vi "点对点.vi"(1 "错误输入":errorcluster, 2 "目标位置":cluster{"x（cm）":dbl, "y（cm）":dbl, "角度（度）":dbl}, 3 "I/O":T11) -> (0 "错误输出":errorcluster)   [LabVIEW 2016]
uses:
  <vilib>/myRIO/Instrument Drivers/Onboard IO/PWM/typedefs/PWM Reference.ctl
  <vilib>/myRIO/Common/Instrument Driver Framework/Utilities/typedefs/myRIO Generic Hardware Reference.ctl
  <vilib>/myRIO/Common/Instrument Driver Framework/Utilities/typedefs/Hardware Version Enum.ctl
  <vilib>/myRIO/Common/Instrument Driver Framework/Utilities/typedefs/myRIO v1.0 Reference.ctl
  <vilib>/myRIO/Common/Instrument Driver Framework/Utilities/typedefs/Generic FPGA Reference.ctl
  <vilib>/myRIO/Common/Instrument Driver Framework/myRIO v1.0/PWM/typedefs/PWM Channels Enum.ctl
  <vilib>/myRIO/Instrument Drivers/Onboard IO/PWM/typedefs/PWM Configuration.ctl
  <vilib>/myRIO/Instrument Drivers/Onboard IO/DIO/typedefs/DIO Reference.ctl
  <vilib>/myRIO/Common/Instrument Driver Framework/myRIO v1.0/DIO/typedefs/DIO Channels List.ctl
  <vilib>/myRIO/Common/Instrument Driver Framework/myRIO v1.0/DIO/typedefs/DIO Channels Enum.ctl
  <vilib>/myRIO/Instrument Drivers/Onboard IO/DIO/DIO.lvlib
  <vilib>/myRIO/Instrument Drivers/Onboard IO/PWM/PWM.lvlib
panel:
  out "前进二":bool
  out "旋转三":bool
  out "旋转二":bool
  out "前进一":bool
  out "速度":dbl[](array[numeric])
  out "旋转一":bool
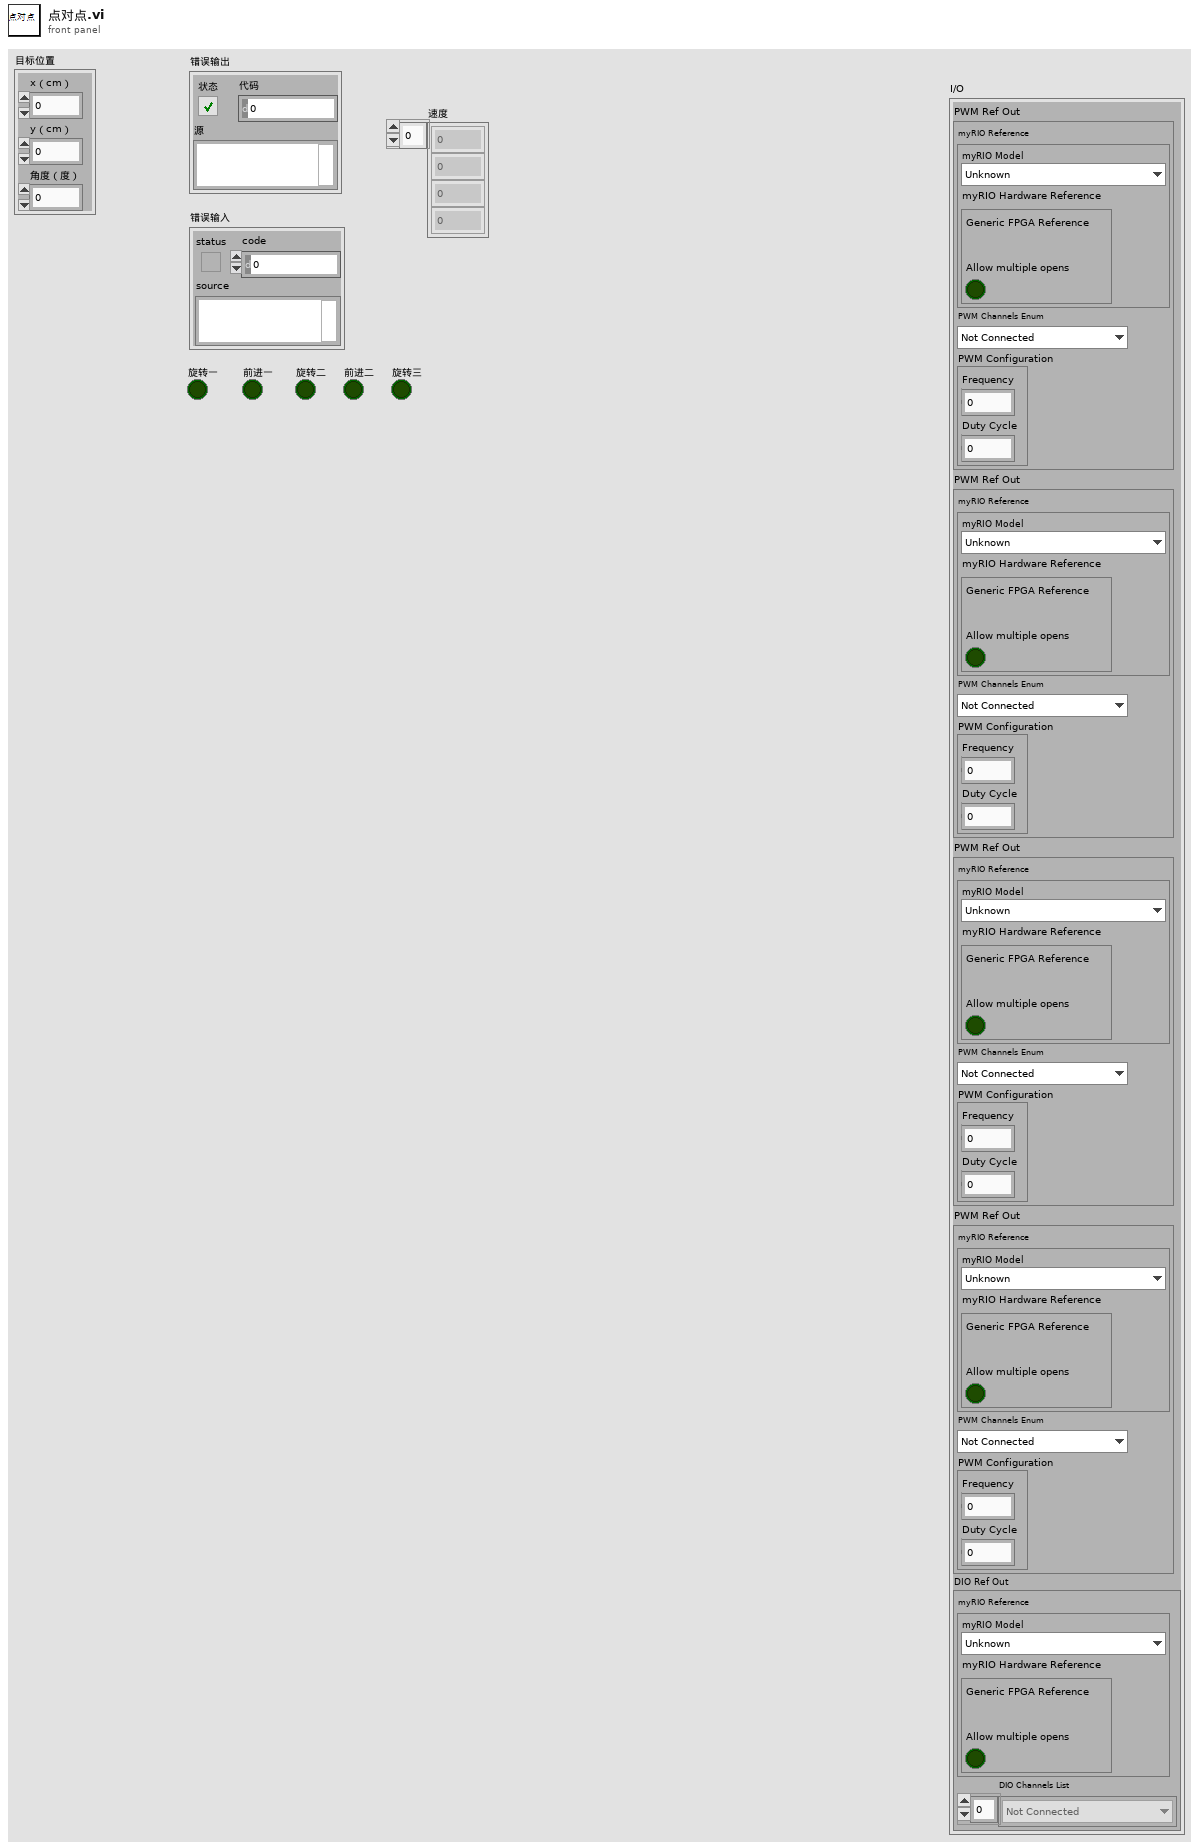
[diagram p1: front panel]
types:
  T1 = typedef "PWM.lvlib/PWM Reference.ctl" = cluster{"myRIO Reference":T2, "PWM Channels Enum":T6, "PWM Configuration":T7}
  T2 = typedef "myRIO Generic Hardware Reference.ctl" = cluster{"myRIO Model":T3, "myRIO Hardware Reference":T4}
  T3 = typedef "Hardware Version Enum.ctl" = enum16{"Unknown", "myRIO-1900", "myRIO-1950", "roboRIO", "NI ELVIS RIO CM"}
  T4 = typedef "myRIO v1.0 Reference.ctl" = cluster{"Generic FPGA Reference":T5, "Allow multiple opens":bool}
  T5 = typedef "Generic FPGA Reference.ctl" = refnum<k20>
  T6 = typedef "PWM Channels Enum.ctl" = enum16{"Not Connected", "C/PWM0", "C/PWM1", "A/PWM0", "A/PWM1", "A/PWM2", "B/PWM0", "B/PWM1", "B/PWM2", "PWM/PWM0", "PWM/PWM1", "PWM/PWM2", "PWM/PWM3", "PWM/PWM4", "PWM/PWM5", "PWM/PWM6", "PWM/PWM7", "PWM/PWM8", "PWM/PWM9"}
  T7 = typedef "PWM.lvlib/PWM Configuration.ctl" = cluster{"Frequency":dbl, "Duty Cycle":dbl}
  T8 = typedef "DIO.lvlib/DIO Reference.ctl" = cluster{"myRIO Reference":T2, "DIO Channels List":T9}
  T9 = typedef "DIO Channels List.ctl" = T10[]
  T10 = typedef "DIO Channels Enum.ctl" = enum16{"Not Connected", "C/DIO0", "C/DIO1", "C/DIO2", "C/DIO3", "C/DIO4", "C/DIO5", "C/DIO6", "C/DIO7", "A/DIO0", "A/DIO1", "A/DIO2", "A/DIO3", "A/DIO4", "A/DIO5", "A/DIO6", "A/DIO7", "A/DIO8", "A/DIO9", "A/DIO10", "A/DIO11", "A/DIO12", "A/DIO13", "A/DIO14", "A/DIO15", "B/DIO0", "B/DIO1", "B/DIO2", "B/DIO3", "B/DIO4", "B/DIO5", "B/DIO6", "B/DIO7", "B/DIO8", "B/DIO9", "B/DIO10", "B/DIO11", "B/DIO12", "B/DIO13", "B/DIO14", "B/DIO15", "LED0", "LED1", "LED2", "LED3", "Button0", "DIO/DIO0", "DIO/DIO1", "DIO/DIO2", "DIO/DIO3", "DIO/DIO4", "DIO/DIO5", "DIO/DIO6", "DIO/DIO7", "DIO/DIO8", "DIO/DIO9", "SPI/CS0", "SPI/CS1", "SPI/CS2", "SPI/CS3", "LED RADIO (Green)", "LED RADIO (Red)", "LED COMM (Green)", "LED COMM (Red)", "LED MODE (Green)", "LED MODE (Red)"}
  T11 = cluster{"PWM Ref Out":T1, "PWM Ref Out":T1, "PWM Ref Out":T1, "PWM Ref Out":T1, "DIO Ref Out":T8}
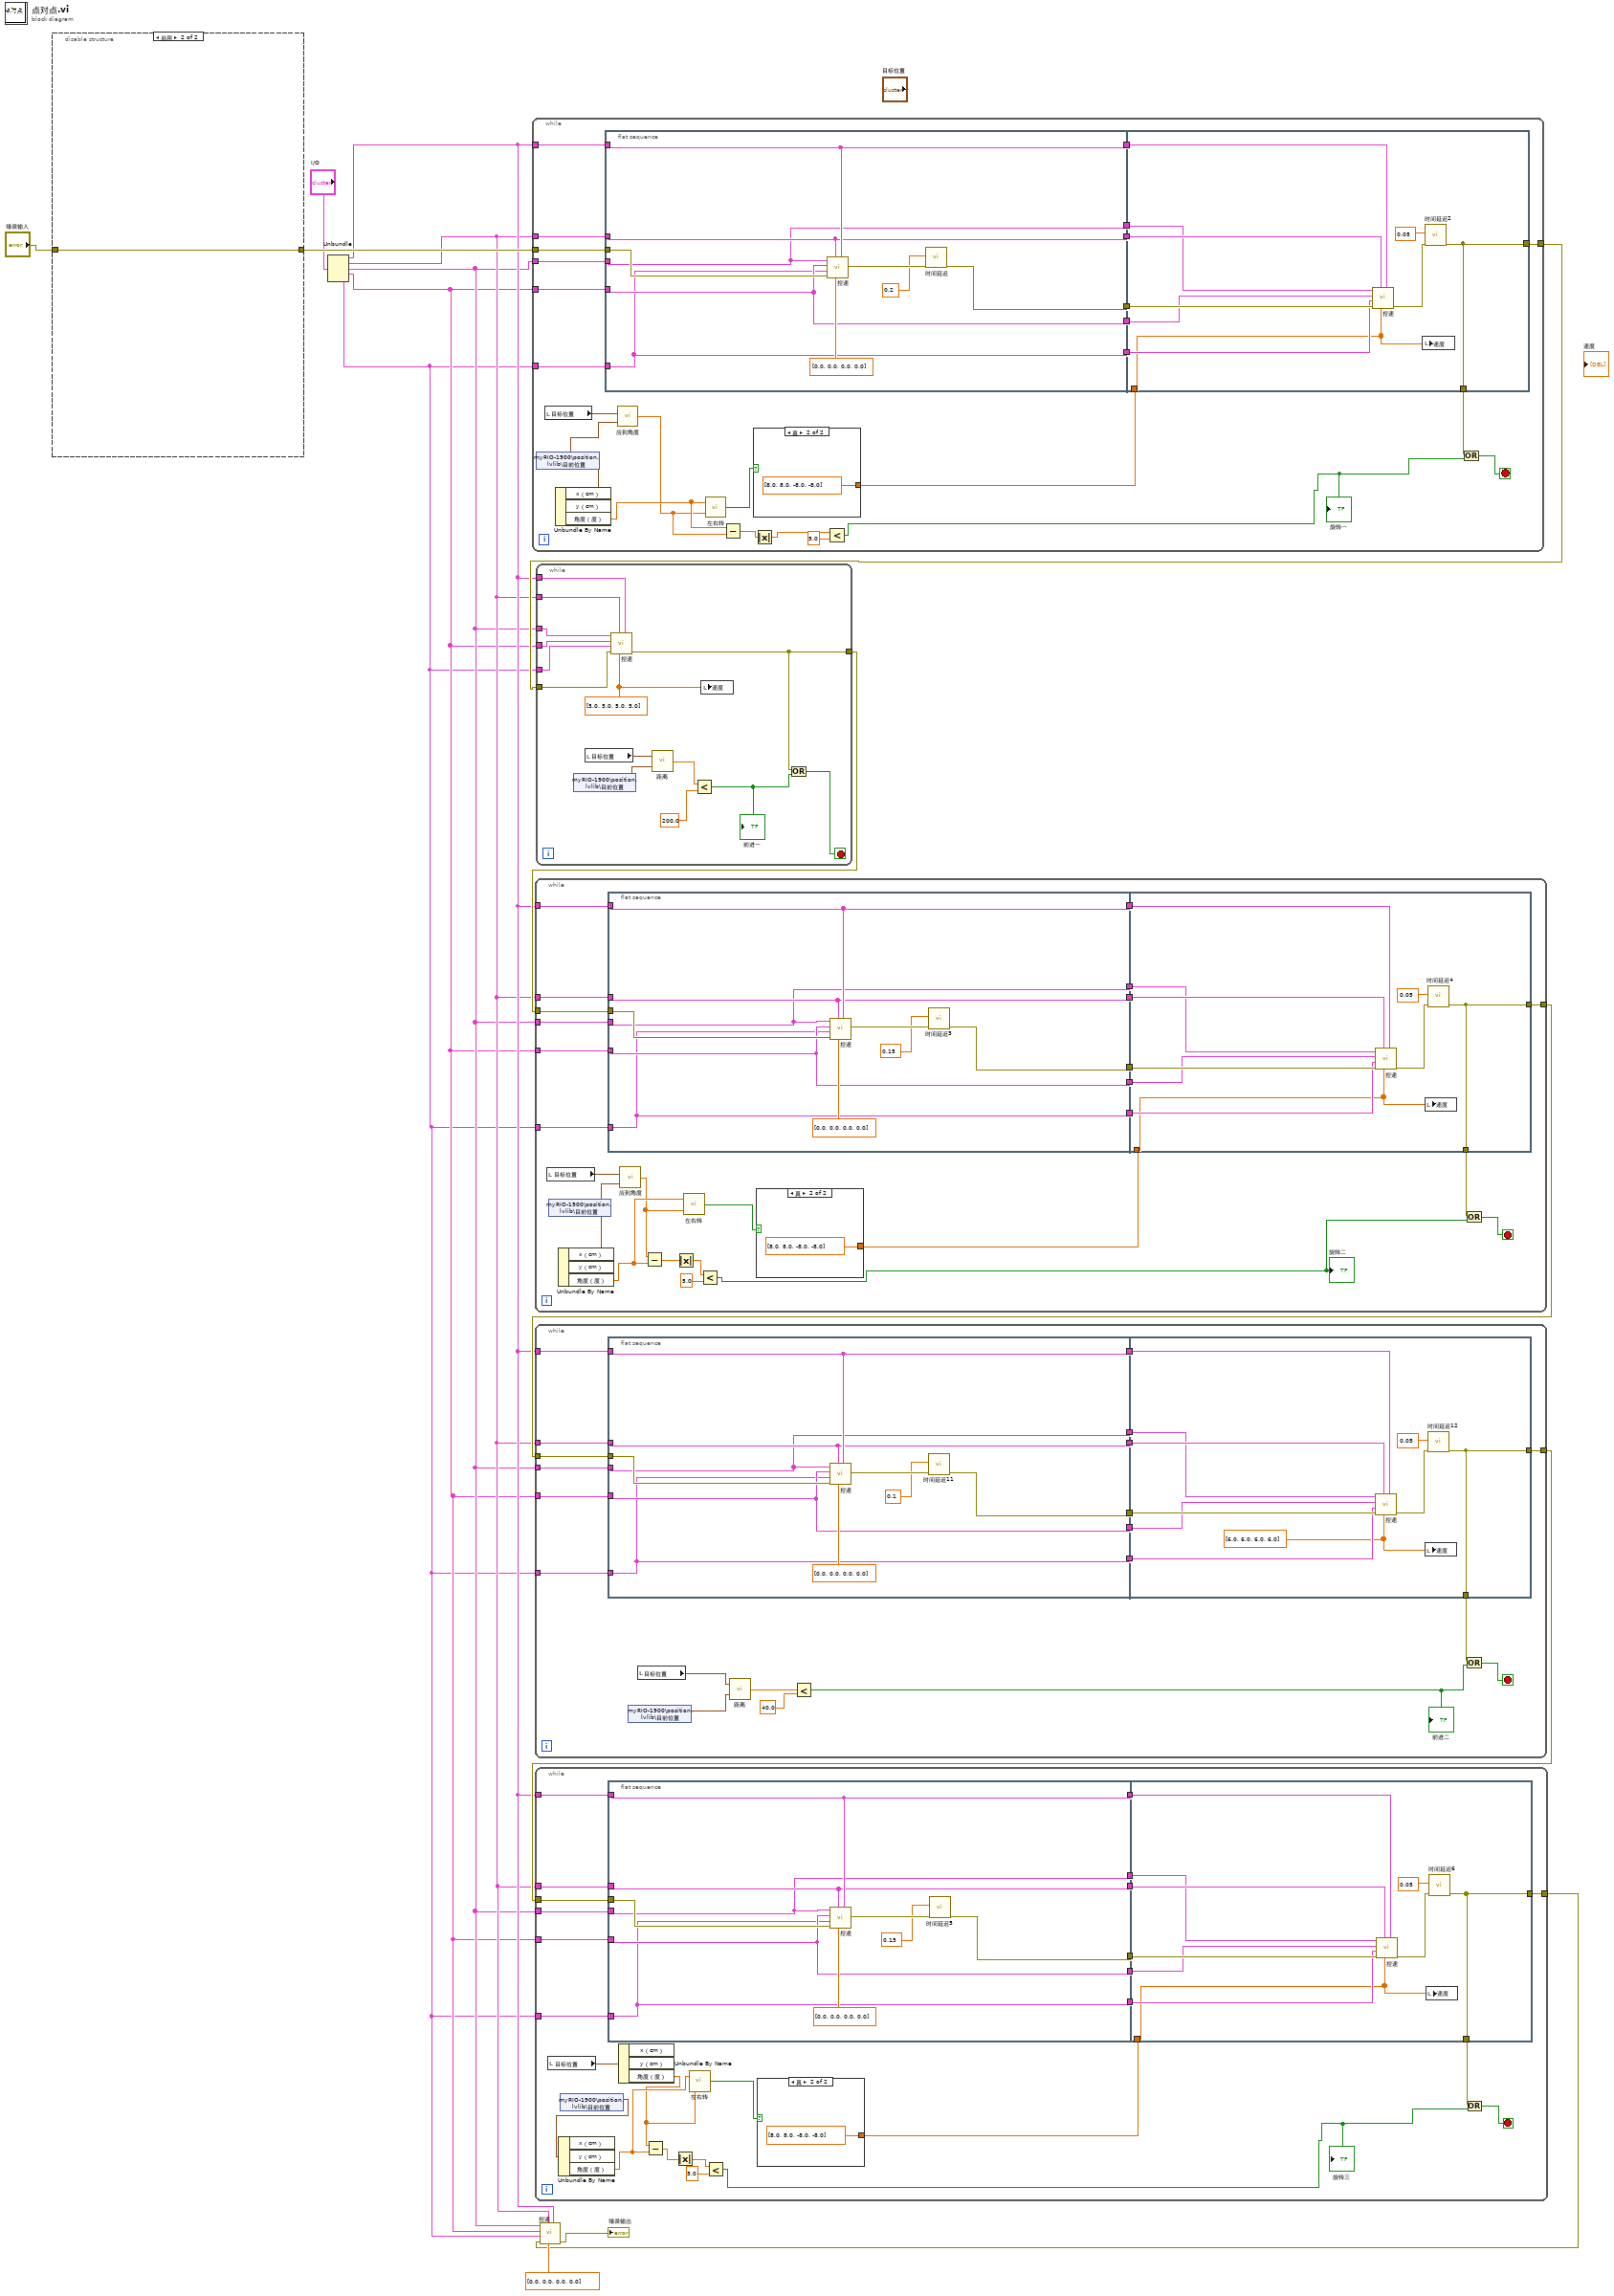
[diagram p0: block diagram]
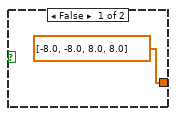
[diagram p2: hidden frame]
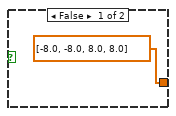
[diagram p3: hidden frame]
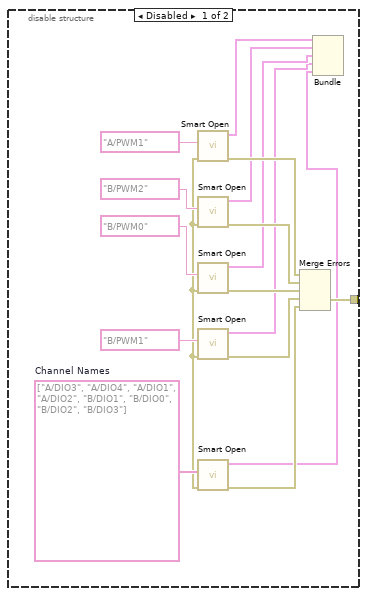
[diagram p4: hidden frame]
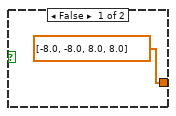
[diagram p5: hidden frame]
diagram:
  n1 = disable-structure shown="启用" {
    disable-tunnel: [w21 w33] -> w15
    disable-tunnel: "错误输入" -> [_ w33]
    frame Disabled {
      w28 = tag[] ["A/DIO3", "A/DIO4", "A/DIO1", "A/DIO2", "B/DIO1", "B/DIO0", "B/DIO2", "B/DIO3"]  # Channel Names
      n2 = call <vilib>:"Smart Open.vi"("Channel Name"=tag "A/PWM1") -> ("error out"=w26:errorcluster, "PWM Ref Out"=w20:T1, "error in (no error)"=w27:errorcluster)  [unwired: 8 in]
      n3 = call <vilib>:"Smart Open.vi"("error in (no error)"=w27, "Channel Name"=tag "B/PWM2") -> ("error out"=w25:errorcluster, "PWM Ref Out"=w19:T1)  [unwired: 8 in]
      n4 = call <vilib>:"Smart Open.vi"("error in (no error)"=w27, "Channel Name"=tag "B/PWM0") -> ("error out"=w24:errorcluster, "PWM Ref Out"=w18:T1)  [unwired: 8 in]
      n5 = call <vilib>:"Smart Open.vi"("error in (no error)"=w27, "Channel Name"=tag "B/PWM1") -> ("error out"=w23:errorcluster, "PWM Ref Out"=w17:T1)  [unwired: 8 in]
      n6 = call <vilib>:"Smart Open.vi"("error in (no error)"=w27, "Channel Names"=w28) -> ("error out"=w22:errorcluster, "DIO Ref Out"=w16:T8)  [unwired: 8 in]
      n7 = Merge Errors(w26, w25, w24, w23, w22) -> (w21:errorcluster)
      n8 = Bundle("PWM Ref Out"=w20, "PWM Ref Out"=w19, "PWM Ref Out"=w18, "PWM Ref Out"=w17, "DIO Ref Out"=w16) -> ()  [unwired: 1 in, 1 out]
    }
    frame Enabled {
    }
  }
  n9 = Unbundle("I/O") -> ("PWM Ref Out"=w8:T1, "PWM Ref Out"=w7:T1, "PWM Ref Out"=w6:T1, "PWM Ref Out"=w5:T1, "DIO Ref Out"=w4:T8)
  n10 = while {
    tunnel: w8 -> [w57]
    tunnel: w7 -> [w56]
    tunnel: w5 -> [w55]
    tunnel: w6 -> [w54]
    tunnel: w15 -> [w53]
    tunnel: w4 -> [w47]
    tunnel: [w45] -> w13
    stop <- w43 stop-if-true
    n11 = shared-variable "myRIO-1900\\position.lvlib\\目前位置"() -> (w41:cluster{"x（cm）":dbl, "y（cm）":dbl, "角度（度）":dbl})  [unwired: 1 in, 1 out]
    n12 = local read "目标位置"() -> (w42:cluster{"x（cm）":dbl, "y（cm）":dbl, "角度（度）":dbl})
    n13 = Unbundle By Name(w41) -> ("角度（度）"=w39:dbl)  [unwired: 2 out]
    n14 = flat-sequence {
      tunnel: w57 -> [w65]
      tunnel: w56 -> [w64]
      tunnel: w55 -> [w62]
      tunnel: w54 -> [w63]
      tunnel: w53 -> [w70]
      tunnel: [w66] -> w52
      tunnel: [w65] -> w51
      tunnel: [w64] -> w50
      tunnel: [w63] -> w49
      tunnel: [w62] -> w48
      tunnel: w47 -> [w61]
      tunnel: [w61] -> w46
      tunnel: w58 -> [w72]
      tunnel: w52 -> [w78]
      tunnel: w51 -> [w77]
      tunnel: w50 -> [w76]
      tunnel: w49 -> [w75]
      tunnel: w48 -> [w74]
      tunnel: w46 -> [w73]
      tunnel: [w71] -> w45
      tunnel: [w71] -> w44
      frame #0 {
        n15 = call "控速.vi"("PWM1"=w65, "速度"=dbl[] [0.0, 0.0, 0.0, 0.0], "PWM2"=w64, "错误输入（无错误）"=w70, "DIO"=w61, "PWM 4"=w62, "PWM 3"=w63) -> ("错误输出"=w68:errorcluster)  [unwired: 4 in]
        n16 = call "时间延迟"("error in (no error)"=w68, "Delay Time (s)"=0.2) -> ("error out"=w66:errorcluster)  [unwired: 9 in]
      }
      frame #1 {
        n17 = call "控速.vi"("PWM1"=w77, "速度"=w72, "PWM2"=w76, "错误输入（无错误）"=w78, "DIO"=w73, "PWM 4"=w74, "PWM 3"=w75) -> ("错误输出"=w80:errorcluster)  [unwired: 4 in]
        n18 = local write "速度"(w72) -> ()
        n19 = call "时间延迟2"("error in (no error)"=w80, "Delay Time (s)"=0.05) -> ("error out"=w71:errorcluster)  [unwired: 9 in]
      }
    }
    n20 = call "应到角度.vi"("目前位置"=w41, "目标位置"=w42) -> ("应到角度"=w38:dbl)
    n21 = call "左右转.vi"("目标角度"=w38, "当前角度"=w39) -> ("左转/右转"=w40:bool)
    n22 = Subtract(x=w39, y=w38) -> (x-y=w37:dbl)
    n23 = case shown="真" w40 {
      tunnel: [dbl[] [-8.0, -8.0, 8.0, 8.0] ("速度") dbl[] [8.0, 8.0, -8.0, -8.0] ("速度")] -> w58
      frame False {
      }
      frame True {
      }
    }
    n24 = Absolute Value(x=w37) -> (abs(x)=w36:dbl)
    n25 = Less?(x=w36, y=5.0) -> (x < y?=w34:bool)
    "旋转一" <- w34
    n26 = Or(x=w44, y=w34) -> (x .or. y?=w43:bool)
  }
  n27 = while {
    tunnel: w8 -> [w94]
    tunnel: w7 -> [w93]
    tunnel: w6 -> [w92]
    tunnel: w5 -> [w91]
    tunnel: w4 -> [w90]
    tunnel: w13 -> [w89]
    tunnel: [w85] -> w12
    stop <- w84 stop-if-true
    w87 = dbl[] [5.0, 5.0, 5.0, 5.0] ("速度")
    n28 = shared-variable "myRIO-1900\\position.lvlib\\目前位置"() -> (w81:cluster{"x（cm）":dbl, "y（cm）":dbl, "角度（度）":dbl})  [unwired: 1 in, 1 out]
    n29 = local read "目标位置"() -> (w82:cluster{"x（cm）":dbl, "y（cm）":dbl, "角度（度）":dbl})
    n30 = call "控速.vi"("PWM1"=w94, "速度"=w87, "PWM2"=w93, "错误输入（无错误）"=w89, "DIO"=w90, "PWM 4"=w91, "PWM 3"=w92) -> ("错误输出"=w85:errorcluster)  [unwired: 4 in]
    n31 = call "距离.vi"("目前位置"=w81, "目标位置"=w82) -> ("距离"=w83:dbl)
    n32 = Less?(x=w83, y=200.0) -> (x < y?=w86:bool)
    "前进一" <- w86
    n33 = local write "速度"(w87) -> ()
    n34 = Or(x=w85, y=w86) -> (x .or. y?=w84:bool)
  }
  n35 = while {
    tunnel: w8 -> [w118]
    tunnel: w7 -> [w117]
    tunnel: w5 -> [w116]
    tunnel: w6 -> [w115]
    tunnel: w12 -> [w114]
    tunnel: w4 -> [w108]
    tunnel: [w106] -> w11
    stop <- w104 stop-if-true
    n36 = local read "目标位置"() -> (w103:cluster{"x（cm）":dbl, "y（cm）":dbl, "角度（度）":dbl})
    n37 = shared-variable "myRIO-1900\\position.lvlib\\目前位置"() -> (w102:cluster{"x（cm）":dbl, "y（cm）":dbl, "角度（度）":dbl})  [unwired: 1 in, 1 out]
    n38 = Unbundle By Name(w102) -> ("角度（度）"=w97:dbl)  [unwired: 2 out]
    n39 = flat-sequence {
      tunnel: w118 -> [w126]
      tunnel: w117 -> [w125]
      tunnel: w116 -> [w123]
      tunnel: w115 -> [w124]
      tunnel: w114 -> [w131]
      tunnel: [w127] -> w113
      tunnel: [w126] -> w112
      tunnel: [w125] -> w111
      tunnel: [w124] -> w110
      tunnel: [w123] -> w109
      tunnel: w108 -> [w122]
      tunnel: [w122] -> w107
      tunnel: w119 -> [w133]
      tunnel: w113 -> [w139]
      tunnel: w112 -> [w138]
      tunnel: w111 -> [w137]
      tunnel: w110 -> [w136]
      tunnel: w109 -> [w135]
      tunnel: w107 -> [w134]
      tunnel: [w132] -> w106
      tunnel: [w132] -> w105
      frame #0 {
        n40 = call "控速.vi"("PWM1"=w126, "速度"=dbl[] [0.0, 0.0, 0.0, 0.0], "PWM2"=w125, "错误输入（无错误）"=w131, "DIO"=w122, "PWM 4"=w123, "PWM 3"=w124) -> ("错误输出"=w129:errorcluster)  [unwired: 4 in]
        n41 = call "时间延迟3"("error in (no error)"=w129, "Delay Time (s)"=0.15) -> ("error out"=w127:errorcluster)  [unwired: 9 in]
      }
      frame #1 {
        n42 = call "控速.vi"("PWM1"=w138, "速度"=w133, "PWM2"=w137, "错误输入（无错误）"=w139, "DIO"=w134, "PWM 4"=w135, "PWM 3"=w136) -> ("错误输出"=w141:errorcluster)  [unwired: 4 in]
        n43 = local write "速度"(w133) -> ()
        n44 = call "时间延迟4"("error in (no error)"=w141, "Delay Time (s)"=0.05) -> ("error out"=w132:errorcluster)  [unwired: 9 in]
      }
    }
    n45 = call "应到角度.vi"("目前位置"=w102, "目标位置"=w103) -> ("应到角度"=w96:dbl)
    n46 = Subtract(x=w96, y=w97) -> (x-y=w101:dbl)
    n47 = Absolute Value(x=w101) -> (abs(x)=w100:dbl)
    n48 = call "左右转.vi"("目标角度"=w96, "当前角度"=w97) -> ("左转/右转"=w95:bool)
    n49 = Less?(x=w100, y=5.0) -> (x < y?=w98:bool)
    "旋转二" <- w98
    n50 = case shown="真" w95 {
      tunnel: [dbl[] [-8.0, -8.0, 8.0, 8.0] ("速度") dbl[] [8.0, 8.0, -8.0, -8.0] ("速度")] -> w119
      frame False {
      }
      frame True {
      }
    }
    n51 = Or(x=w105, y=w98) -> (x .or. y?=w104:bool)
  }
  n52 = while {
    tunnel: w8 -> [w161]
    tunnel: w7 -> [w160]
    tunnel: w5 -> [w159]
    tunnel: w6 -> [w158]
    tunnel: w11 -> [w157]
    tunnel: w4 -> [w151]
    tunnel: [w149] -> w10
    stop <- w147 stop-if-true
    n53 = flat-sequence {
      tunnel: w161 -> [w166]
      tunnel: w160 -> [w165]
      tunnel: w159 -> [w163]
      tunnel: w158 -> [w164]
      tunnel: w157 -> [w171]
      tunnel: [w167] -> w156
      tunnel: [w166] -> w155
      tunnel: [w165] -> w154
      tunnel: [w164] -> w153
      tunnel: [w163] -> w152
      tunnel: w151 -> [w162]
      tunnel: [w162] -> w150
      tunnel: w156 -> [w179]
      tunnel: w155 -> [w178]
      tunnel: w154 -> [w177]
      tunnel: w153 -> [w176]
      tunnel: w152 -> [w175]
      tunnel: w150 -> [w174]
      tunnel: [w173] -> w149
      tunnel: [w173] -> w148
      frame #0 {
        n54 = call "控速.vi"("PWM1"=w166, "速度"=dbl[] [0.0, 0.0, 0.0, 0.0], "PWM2"=w165, "错误输入（无错误）"=w171, "DIO"=w162, "PWM 4"=w163, "PWM 3"=w164) -> ("错误输出"=w169:errorcluster)  [unwired: 4 in]
        n55 = call "时间延迟11"("error in (no error)"=w169, "Delay Time (s)"=0.1) -> ("error out"=w167:errorcluster)  [unwired: 9 in]
      }
      frame #1 {
        w172 = dbl[] [6.0, 6.0, 6.0, 6.0] ("速度")
        n56 = call "控速.vi"("PWM1"=w178, "速度"=w172, "PWM2"=w177, "错误输入（无错误）"=w179, "DIO"=w174, "PWM 4"=w175, "PWM 3"=w176) -> ("错误输出"=w181:errorcluster)  [unwired: 4 in]
        n57 = local write "速度"(w172) -> ()
        n58 = call "时间延迟12"("error in (no error)"=w181, "Delay Time (s)"=0.05) -> ("error out"=w173:errorcluster)  [unwired: 9 in]
      }
    }
    n59 = shared-variable "myRIO-1900\\position.lvlib\\目前位置"() -> (w145:cluster{"x（cm）":dbl, "y（cm）":dbl, "角度（度）":dbl})  [unwired: 1 in, 1 out]
    n60 = local read "目标位置"() -> (w146:cluster{"x（cm）":dbl, "y（cm）":dbl, "角度（度）":dbl})
    n61 = call "距离.vi"("目前位置"=w145, "目标位置"=w146) -> ("距离"=w144:dbl)
    n62 = Less?(x=w144, y=40.0) -> (x < y?=w142:bool)
    "前进二" <- w142
    n63 = Or(x=w148, y=w142) -> (x .or. y?=w147:bool)
  }
  n64 = while {
    tunnel: w8 -> [w205]
    tunnel: w7 -> [w204]
    tunnel: w5 -> [w203]
    tunnel: w6 -> [w202]
    tunnel: w10 -> [w201]
    tunnel: w4 -> [w195]
    tunnel: [w193] -> w2
    stop <- w191 stop-if-true
    n65 = local read "目标位置"() -> (w190:cluster{"x（cm）":dbl, "y（cm）":dbl, "角度（度）":dbl})
    n66 = shared-variable "myRIO-1900\\position.lvlib\\目前位置"() -> (w189:cluster{"x（cm）":dbl, "y（cm）":dbl, "角度（度）":dbl})  [unwired: 1 in, 1 out]
    n67 = Unbundle By Name(w189) -> ("角度（度）"=w188:dbl)  [unwired: 2 out]
    n68 = flat-sequence {
      tunnel: w205 -> [w213]
      tunnel: w204 -> [w212]
      tunnel: w203 -> [w210]
      tunnel: w202 -> [w211]
      tunnel: w201 -> [w218]
      tunnel: [w214] -> w200
      tunnel: [w213] -> w199
      tunnel: [w212] -> w198
      tunnel: [w211] -> w197
      tunnel: [w210] -> w196
      tunnel: w195 -> [w209]
      tunnel: [w209] -> w194
      tunnel: w206 -> [w220]
      tunnel: w200 -> [w226]
      tunnel: w199 -> [w225]
      tunnel: w198 -> [w224]
      tunnel: w197 -> [w223]
      tunnel: w196 -> [w222]
      tunnel: w194 -> [w221]
      tunnel: [w219] -> w193
      tunnel: [w219] -> w192
      frame #0 {
        n69 = call "控速.vi"("PWM1"=w213, "速度"=dbl[] [0.0, 0.0, 0.0, 0.0], "PWM2"=w212, "错误输入（无错误）"=w218, "DIO"=w209, "PWM 4"=w210, "PWM 3"=w211) -> ("错误输出"=w216:errorcluster)  [unwired: 4 in]
        n70 = call "时间延迟5"("error in (no error)"=w216, "Delay Time (s)"=0.15) -> ("error out"=w214:errorcluster)  [unwired: 9 in]
      }
      frame #1 {
        n71 = call "控速.vi"("PWM1"=w225, "速度"=w220, "PWM2"=w224, "错误输入（无错误）"=w226, "DIO"=w221, "PWM 4"=w222, "PWM 3"=w223) -> ("错误输出"=w228:errorcluster)  [unwired: 4 in]
        n72 = local write "速度"(w220) -> ()
        n73 = call "时间延迟6"("error in (no error)"=w228, "Delay Time (s)"=0.05) -> ("error out"=w219:errorcluster)  [unwired: 9 in]
      }
    }
    n74 = Unbundle By Name(w190) -> ("角度（度）"=w187:dbl)  [unwired: 2 out]
    n75 = Subtract(x=w187, y=w188) -> (x-y=w186:dbl)
    n76 = Absolute Value(x=w186) -> (abs(x)=w185:dbl)
    n77 = call "左右转.vi"("目标角度"=w187, "当前角度"=w188) -> ("左转/右转"=w183:bool)
    n78 = Less?(x=w185, y=5.0) -> (x < y?=w182:bool)
    "旋转三" <- w182
    n79 = case shown="真" w183 {
      tunnel: [dbl[] [-8.0, -8.0, 8.0, 8.0] ("速度") dbl[] [8.0, 8.0, -8.0, -8.0] ("速度")] -> w206
      frame False {
      }
      frame True {
      }
    }
    n80 = Or(x=w192, y=w182) -> (x .or. y?=w191:bool)
  }
  n81 = call "控速.vi"("PWM1"=w8, "速度"=dbl[] [0.0, 0.0, 0.0, 0.0], "PWM2"=w7, "错误输入（无错误）"=w2, "DIO"=w4, "PWM 4"=w5, "PWM 3"=w6) -> ("错误输出"=→"错误输出":errorcluster)  [unwired: 4 in]
